vi "data_change_detection.vi"(10 "input_data":dbl) -> (2 "detection":bool)   [LabVIEW 2020]
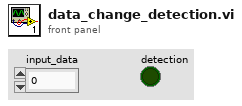
[diagram p1: front panel]
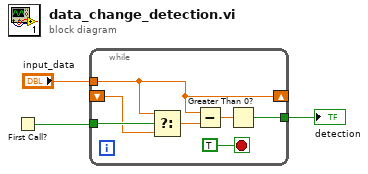
[diagram p0: block diagram]
diagram:
  n1 = First Call?() -> (First Call?: T/F=w1:bool)
  n2 = while {
    shift-right: [w6] -> _
    shift-left: _ -> [w4]
    tunnel: [w8] -> w3
    tunnel: "input_data" -> [w6]
    tunnel: w1 -> [w7]
    stop <- TRUE stop-if-true
    n3 = Select(t=w6, s=w7, f=w4) -> (s? t:f=w5:dbl)
    n4 = Subtract(x=w6, y=w5) -> (x-y=w9:dbl)
    n5 = Greater Than 0?(x=w9) -> (x > 0?=w8:bool)
  }
  "detection" <- w3
